vi "Global 2.vi"() -> ()   [LabVIEW 2020]
panel:
  out "Numeric":dbl
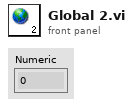
[diagram p1: front panel]
diagram:
